vi "write_params.vi"(8 "error in (no error)":errorcluster, 10 "params":T1={"threshold"=0.5, "branching_factor"=50, "n_clusters"=3.0, "compute_labels"=TRUE, "copy"=TRUE}, 11 "Birch in":refnum<class "Birch.lvclass">) -> (0 "error out":errorcluster, 3 "Birch out":refnum<class "Birch.lvclass">)   [LabVIEW 2020, in "Birch.lvclass"]
uses:
  Birch.lvclass
  Controls/birch_params.ctl
  Birch.lvclass/Birch.ctl
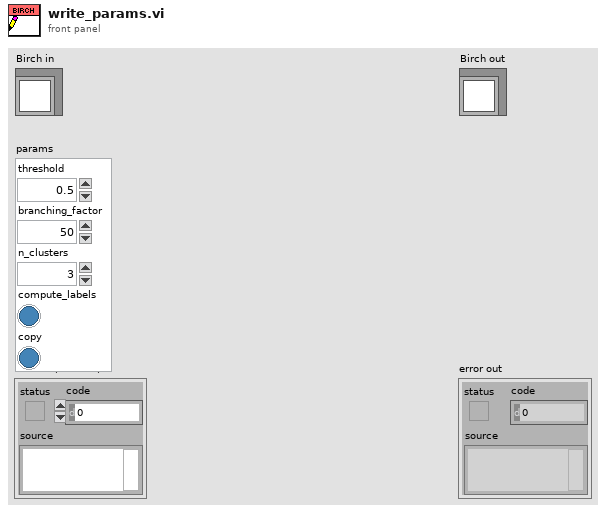
[diagram p1: front panel]
types:
  T1 = typedef "birch_params.ctl" = cluster{"threshold":dbl, "branching_factor":i32, "n_clusters":dbl, "compute_labels":bool, "copy":bool}
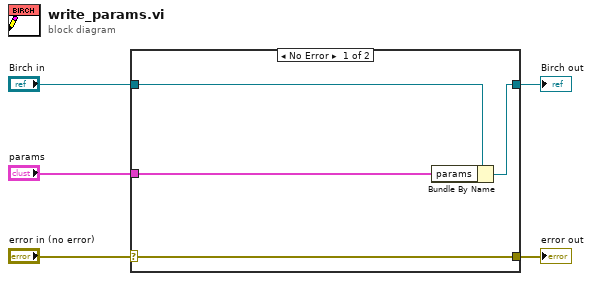
[diagram p0: block diagram]
diagram:
  n1 = case shown="No Error" "error in (no error)" {
    selector: "error in (no error)" -> [w9 w10]
    tunnel: [w9 w10] -> w4
    tunnel: [w7 w11] -> w2
    tunnel: "Birch in" -> [w8 w11]
    tunnel: "params" -> [w6 _]
    frame No Error {
      n2 = Bundle By Name(cluster=w8, "params"=w6) -> (w7:refnum<class "Birch.lvclass">)
    }
    frame Error {
    }
  }
  "error out" <- w4
  "Birch out" <- w2
